vi "DAQmx-AI.DVRtoRef.vi"(10 "Ref":T1) -> (2 "Ref":u32 format="%08x")   [LabVIEW 2016, in "DAQmx-AI.lvclass"]
doc: "JKI State Machine Objects (SMO) 1.0.0.5\nJKI - JKI\nCopyright (c) 2016, JKI"
uses:
  DAQmx-AI.lvclass
  Typedefs/PrivateData--Ref.ctl
  Typedefs/PrivateData--Cluster.ctl
  Typedefs/Configuration--Cluster.ctl
  Typedefs/Units -- Enum.ctl
  Typedefs/PublicEvents--Cluster.ctl
  Typedefs/DataChanged--EventData--Cluster.ctl
  Typedefs/ScalingEvent--Cluster.ctl
  Typedefs/Scaling(MapRange)--Cluster.ctl
  Typedefs/Scaling--Cluster.ctl
  Typedefs/ScalingType--Enum.ctl
  Typedefs/Scaling(Linear)--Cluster.ctl
  Typedefs/Scaling(Polynomial)--Cluster.ctl
  Typedefs/Scaling(Table)--Cluster.ctl
  Typedefs/PrivateEvents--Cluster.ctl
  Typedefs/Logging--Cluster.ctl
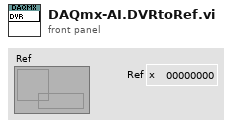
[diagram p1: front panel]
types:
  T1 = typedef "DAQmx-AI.lvclass/PrivateData--Ref.ctl" = refnum<data-value>
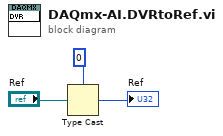
[diagram p0: block diagram]
diagram:
  n1 = Type Cast(type=u32 0 ("Ref"), x="Ref") -> (*(type *) &x=→"Ref":u32)
